vi "Test Get Summary of Case.vi"(8 "error in (no error)":errorcluster, 11 "Result Model Result Recording Test in":refnum<class "Result Model Result Recording Test.lvclass">) -> (0 "error out":errorcluster, 3 "Result Model Result Recording Test out":refnum<class "Result Model Result Recording Test.lvclass">)   [LabVIEW 2020, in "Result Model Result Recording Test.lvclass"]
uses:
  Result Model Result Recording Test.lvclass
  source/Core/Result/Type.ctl
  source/Core/Result/Result.lvlib
  source/Core/Result/Status.ctl
  source/Core/Result/Result.ctl
  source/User Interface/Result Model/Result Model.lvclass
  <vilib>/Astemes/LUnit/Palette/Advanced Assertions/LUnit Advanced Assertions.lvlib
  C:/Program Files (x86)/National Instruments/LabVIEW 2020/vi.lib/Astemes/LUnit/Test Case.lvclass
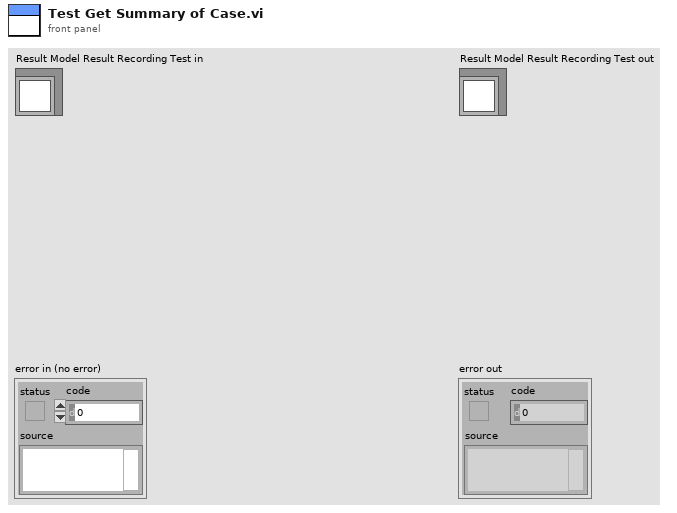
[diagram p1: front panel]
types:
  T1 = typedef "Result.lvlib/Result.ctl" = cluster{"Name":string, "Description":string, "Status":T2, "Result Type":T3, "Execution Time":dbl, "Data":cluster{"Expected":variant, "Actual":variant, "Delta":variant}}
  T2 = typedef "Result.lvlib/Status.ctl" = enum16{"", "Passed", "Failed", "Error", "Skipped", "Setup Error", "Broken", "Teardown Error"}
  T3 = typedef "Result.lvlib/Type.ctl" = enum16{"Test Case", "Test Suite", "Test Run", "Pass", "Fail", "Skip", "Pass if", "Fail if", "Pass if Error", "Fail if Error", "Pass if Equal", "Fail if Equal"}
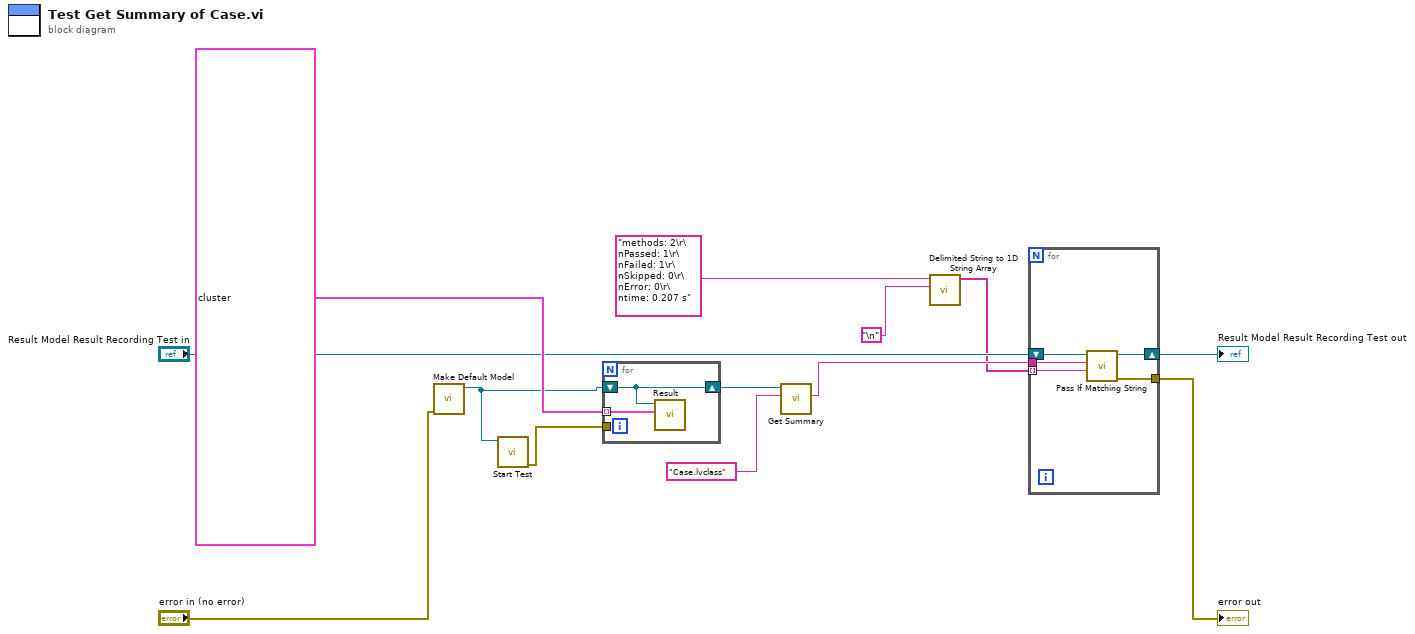
[diagram p0: block diagram]
diagram:
  n1 = call "Make Default Model.vi"("error in (no error)"="error in (no error)") -> ("Result Model out"=w5:refnum<class "Result Model.lvclass">)  [unwired: 9 in, 1 out]
  n2 = call "Start Test.vi"("Result Model by Reference In"=w5) -> ("error out"=w4:errorcluster)  [unwired: 10 in]
  n3 = for {
    tunnel: T1[] [{"Name"="Case.lvclass:Test Method.vi", "Description"="Passed:\nMessage", "Status"=enum."Passed", "Result Type"=enum."Test Case", "Execution Time"=0.107, "Data"={"Expected"=variant, "Actual"=variant, "Delta"=variant}}, {"Name"="Case.lvclass:Test Method2.vi", "Description"="", "Status"=enum."Failed", "Result Type"=enum."Test Case", "Execution Time"=0.1, "Data"={"Expected"=variant, "Actual"=variant, "Delta"=variant}}, {"Name"="Case.lvclass", "Description"="", "Status"=enum."Failed", "Result Type"=enum."Test Suite", "Execution Time"=0.0, "Data"={"Expected"=variant, "Actual"=variant, "Delta"=variant}}] ("Results") -> [w15] mode=indexing
    shift-right: [w14] -> w8
    shift-left: w5 -> [w14]
    tunnel: w4 -> [_]
    n4 = call-dynamic "Result.vi"("Results"=w15, "Result Model by Reference In"=w14) -> ()  [unwired: 9 in, 1 out]
  }
  n5 = call "Get Summary.vi"("Item"="Case.lvclass", "Result Model by Reference In"=w8) -> ("Summary"=w6:string)  [unwired: 8 in, 1 out]
  n6 = call <vilib>:"Delimited String to 1D String Array.vi"("delimiter"="\n", "delimited string"="methods: 2\r\nPassed: 1\r\nFailed: 1\r\nSkipped: 0\r\nError: 0\r\ntime: 0.207 s") -> ("string array"=w1:string[])  [unwired: 9 in]
  n7 = for {
    tunnel: [w18] -> w10
    tunnel: w6 -> [w17]
    shift-right: [w19] -> w11
    shift-left: "Result Model Result Recording Test in" -> [w20]
    tunnel: w1 -> [w16] mode=indexing
    n8 = call <vilib>:"Pass If Matching String.vi"("Regular Expression"=w16, "String"=w17, "LUnit Test Case In"=w20) -> ("error out"=w18:errorcluster, "LUnit Test Case Out"=w19:refnum<class "Result Model Result Recording Test.lvclass">)  [unwired: 7 in]
  }
  "error out" <- w10
  "Result Model Result Recording Test out" <- w11
